vi "(auto) Go back controller.vi"(10 "CurDot":T1(ring), 11 "BackStates":enum16{"0", "1", "2", "3", "4", "5", "6", ""}(ring)) -> (3 "BackState out":enum16{"0", "1", "2", "3", "4", "5", "6", ""}(ring))   [LabVIEW 2017]
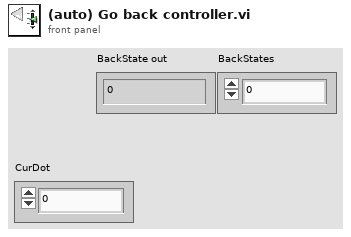
[diagram p1: front panel]
types:
  T1 = enum16{"0", "1", "2", "3", "4", "5", "6", "7", "8", "9", "10", "11", "12", "13", "14", "15", "16", "17", "18", "19", "20", "21", "22", "23", "24", "25", "26", "27", "28", "29", "30", "31", "32", "33", "34", "35"}
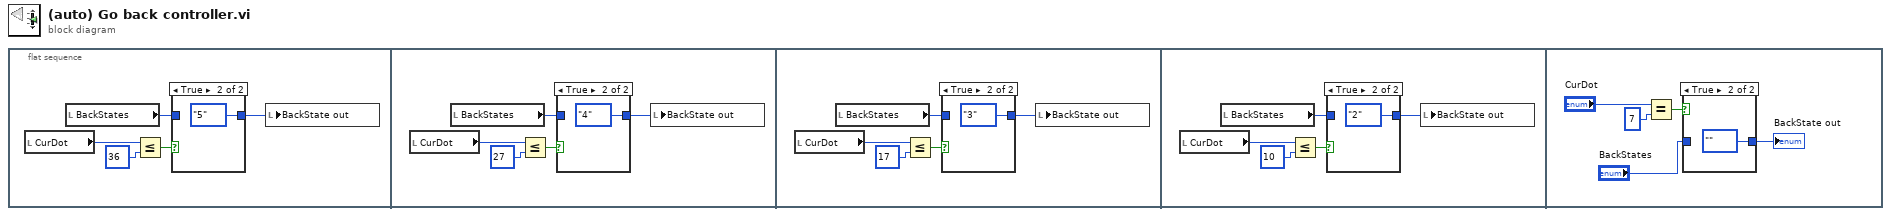
[diagram p0: block diagram]
diagram:
  n1 = flat-sequence {
    frame #0 {
      n2 = local read "CurDot"() -> (w3:T1)
      n3 = local read "BackStates"() -> (w4:enum16{"0", "1", "2", "3", "4", "5", "6", ""})
      n4 = Less Or Equal?(x=w3, y=36) -> (x <= y?=w5:bool)
      n5 = case shown="True" w5 {
        tunnel: [w6 enum16{"0", "1", "2", "3", "4", "5", "6", ""}."5" ("BackStates out")] -> w2
        tunnel: w4 -> [w6 _]
        frame False {
        }
        frame True {
        }
      }
      n6 = local write "BackState out"(w2) -> ()
    }
    frame #1 {
      n7 = local read "CurDot"() -> (w10:T1)
      n8 = local read "BackStates"() -> (w11:enum16{"0", "1", "2", "3", "4", "5", "6", ""})
      n9 = Less Or Equal?(x=w10, y=27) -> (x <= y?=w12:bool)
      n10 = case shown="True" w12 {
        tunnel: [w13 enum16{"0", "1", "2", "3", "4", "5", "6", ""}."4" ("BackStates out")] -> w9
        tunnel: w11 -> [w13 _]
        frame False {
        }
        frame True {
        }
      }
      n11 = local write "BackState out"(w9) -> ()
    }
    frame #2 {
      n12 = local read "CurDot"() -> (w17:T1)
      n13 = local read "BackStates"() -> (w18:enum16{"0", "1", "2", "3", "4", "5", "6", ""})
      n14 = Less Or Equal?(x=w17, y=17) -> (x <= y?=w19:bool)
      n15 = case shown="True" w19 {
        tunnel: [w20 enum16{"0", "1", "2", "3", "4", "5", "6", ""}."3" ("BackStates out")] -> w16
        tunnel: w18 -> [w20 _]
        frame False {
        }
        frame True {
        }
      }
      n16 = local write "BackState out"(w16) -> ()
    }
    frame #3 {
      n17 = local read "CurDot"() -> (w26:T1)
      n18 = local read "BackStates"() -> (w25:enum16{"0", "1", "2", "3", "4", "5", "6", ""})
      n19 = Less Or Equal?(x=w26, y=10) -> (x <= y?=w24:bool)
      n20 = case shown="True" w24 {
        tunnel: [w27 enum16{"0", "1", "2", "3", "4", "5", "6", ""}."2" ("BackStates out")] -> w23
        tunnel: w25 -> [w27 _]
        frame False {
        }
        frame True {
        }
      }
      n21 = local write "BackState out"(w23) -> ()
    }
    frame #4 {
      n22 = Equal?(x="CurDot", y=7) -> (x = y?=w31:bool)
      n23 = case shown="True" w31 {
        tunnel: [w34 enum16{"0", "1", "2", "3", "4", "5", "6", ""}."" ("BackStates out")] -> w32
        tunnel: "BackStates" -> [w34 _]
        frame False {
        }
        frame True {
        }
      }
      "BackState out" <- w32
    }
  }
